vi "Optimized Particle Score v2.vi"() -> ()   [LabVIEW 2012]
uses:
  <vilib>/vision/Image Controls.llb/IMAQ Image.ctl
  <vilib>/vision/NI_Vision_Development_Module.lvlib
panel:
  in  "Particle Count Limit":i32=2147483647
  in  "Area Size Limit":dbl
  out "Sorted Data":dbl[][](array[numeric])
  in  "Pixel Measurements":T1[](array[typedef])=[35, 4, 5, 6, 7] items=["Center of Mass X", "Center of Mass Y", "First Pixel X", "First Pixel Y", "Bounding Rect Left", "Bounding Rect Top", "Bounding Rect Right", "Bounding Rect Bottom", "Max Feret Diameter Start X", "Max Feret Diameter Start Y", "Max Feret Diameter End X", "Max Feret Diameter End Y", "Max Horiz. Segment Length Left", "Max Horiz. Segment Length Right", "Max Horiz. Segment Length Row", "-", "Bounding Rect Width", "Bounding Rect Height", "Bounding Rect Diagonal", "Perimeter", "Convex Hull Perimeter", "Holes' Perimeter", "Max Feret Diameter", "Equivalent Ellipse Major Axis", "Equivalent Ellipse Minor Axis", "Equivalent Ellipse Minor Axis (Feret)", "Equivalent Rect Long Side", "Equivalent Rect Short Side", "Equivalent Rect Diagonal", "Equivalent Rect Short Side (Feret)", "Average Horiz. Segment Length", "Average Vert. Segment Length", "Hydraulic Radius", "Waddel Disk Diameter", "-", "Area", "Holes' Area", "Particle & Holes' Area", "Convex Hull Area", "Image Area", "-", "Number of Holes", "Number of Horiz. Segments", "Number of Vert. Segments", "-", "Orientation", "Max Feret Diameter Orientation", "-", "% Area/Image Area", "% Area/(Particle & Holes' Area)", "Ratio of Equivalent Ellipse Axes", "Ratio of Equivalent Rect Sides", "-", "Elongation Factor", "Compactness Factor", "Heywood Circularity Factor", "Type Factor", "-", "Sum X", "Sum Y", "Sum XX", "Sum XY", "Sum YY", "Sum XXX", "Sum XXY", "Sum XYY", "Sum YYY", "-", "Moment of Inertia XX", "Moment of Inertia XY", "Moment of Inertia YY", "Moment of Inertia XXX", "Moment of Inertia XXY", "Moment of Inertia XYY", "Moment of Inertia YYY", "Norm. Moment of Inertia XX", "Norm. Moment of Inertia XY", "Norm. Moment of Inertia YY", "Norm. Moment of Inertia XXX", "Norm. Moment of Inertia XXY", "Norm. Moment of Inertia XYY", "Norm. Moment of Inertia YYY", "Hu Moment 1", "Hu Moment 2", "Hu Moment 3", "Hu Moment 4", "Hu Moment 5", "Hu Moment 6", "Hu Moment 7"]
  out "Particles":i32
  in  "Image in":T2
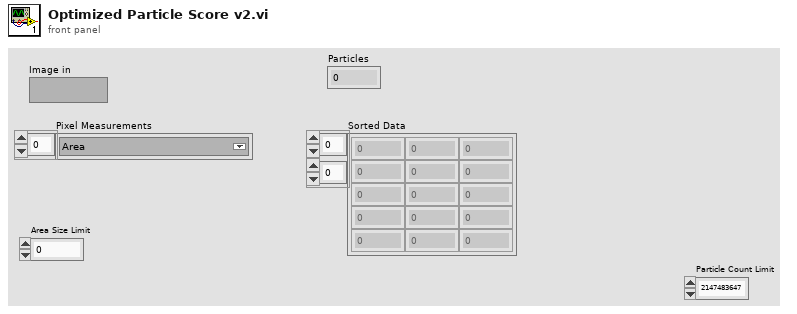
[diagram p1: front panel]
types:
  T1 = typedef "Particle Parameters" = i32
  T2 = typedef "IMAQ Image.ctl" = refnum<image>
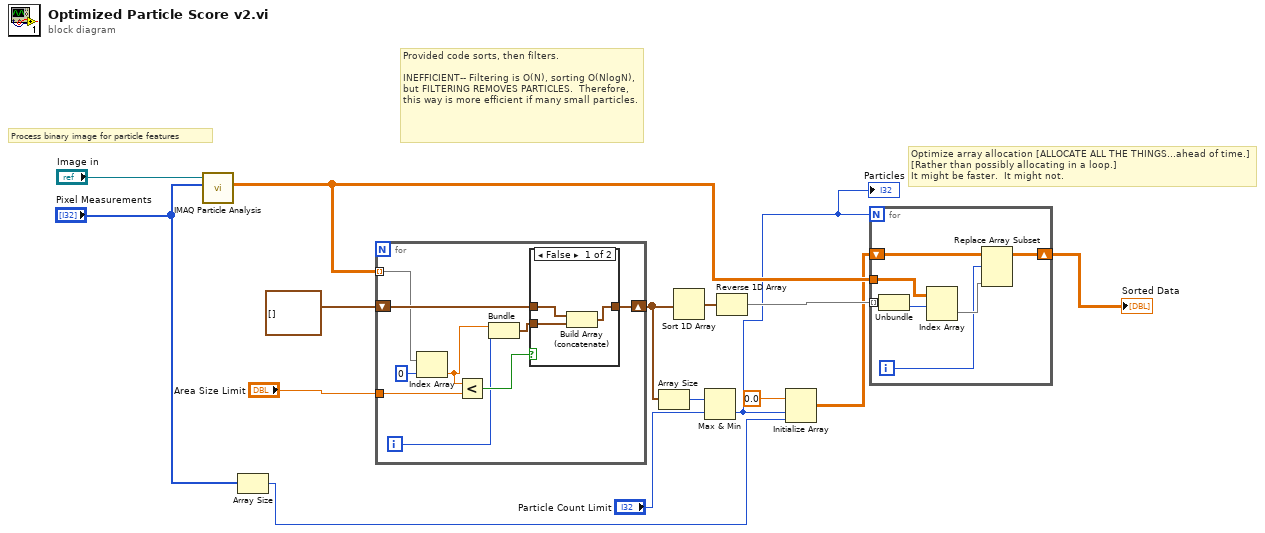
[diagram p0: block diagram]
diagram:
  # "Optimize array allocation [ALLOCATE ALL THE THINGS...ahead of time.]\n[Rather than possibly allocating in a loop.]\nIt might be faster.  It might not."
  # "Provided code sorts, then filters.\n\nINEFFICIENT-- Filtering is O(N), sorting O(NlogN),\nbut FILTERING REMOVES PARTICLES.  Therefore, this way is more efficient if many small particles."
  # "Process binary image for particle features"
  n1 = call "IMAQ Particle Analysis"("Pixel Measurements"="Pixel Measurements", "Image"="Image in") -> ("Particle Measurements (Pixels)"=w3:dbl[][])  [unwired: 3 in, 6 out]
  n2 = Array Size(array="Pixel Measurements") -> (size(s)=w7:i32)
  n3 = for {
    tunnel: w3 -> [w20] mode=indexing
    shift-right: [w23] -> w5
    shift-left: cluster{"Numeric":dbl, i32}[] [] -> [w24]
    tunnel: "Area Size Limit" -> [w22]
    i -> [w16]
    n4 = Index Array(array=w20, index=0) -> (element=w18:dbl)
    n5 = Less?(x=w18, y=w22) -> (x < y?=w21:bool)
    n6 = Bundle("Numeric"=w18, w16) -> (w17:cluster{"Numeric":dbl, i32})  [unwired: 1 in]
    n7 = case shown="False" w21 {
      tunnel: w24 -> [w27 w28]
      tunnel: [w26 w28] -> w23
      tunnel: w17 -> [w25 _]
      frame False {
        n8 = Build Array (concatenate)(w27, w25) -> (w26:cluster{"Numeric":dbl, i32}[])
      }
      frame True {
      }
    }
  }
  n9 = Array Size(array=w5) -> (size(s)=w4:i32)
  n10 = Sort 1D Array(array=w5) -> (sorted array=w13:cluster{"Numeric":dbl, i32}[])
  n11 = Max & Min(x=w4, y="Particle Count Limit") -> (min(x,y)=w2:i32)  [unwired: 1 out]
  "Particles" <- w2
  n12 = Reverse 1D Array(array=w13) -> (reversed array=w11:cluster{"Numeric":dbl, i32}[])
  n13 = Initialize Array(0.0, w2, w7) -> (w1:dbl[][])
  n14 = for {
    N: w2 -> [_]
    tunnel: w11 -> [w35] mode=indexing
    shift-right: [w29] -> w10
    shift-left: w1 -> [w32]
    tunnel: w3 -> [w33]
    i -> [w30]
    n15 = Unbundle(w35) -> (w34:i32)  [unwired: 1 out]
    n16 = Index Array(array=w33, index (row)=w34) -> (element=w31:dbl[])  [unwired: 1 in]
    n17 = Replace Array Subset(array=w32, new element=w31, index (row)=w30) -> (w29:dbl[][])  [unwired: 1 in]
  }
  "Sorted Data" <- w10
